vi "Read_queue_data.vi"(0 "Queue DVR in":refnum<data-value>, 11 "error in (no error)":errorcluster) -> (4 "Queue DVR out":refnum<data-value>, 6 "DATA":T1, 15 "error out":errorcluster)   [LabVIEW 2020, in "Data Communication Transmitter.lvlib" / "Queue.lvclass"]
uses:
  Classes/Children/Intra-Application/Children/With Data/Children/Queues/Queue.lvclass
  Classes/Children/Intra-Application/Children/With Data/Children/Queues/Queue.lvclass/Queue.ctl
  Accessors/Read/Read DATA.vi
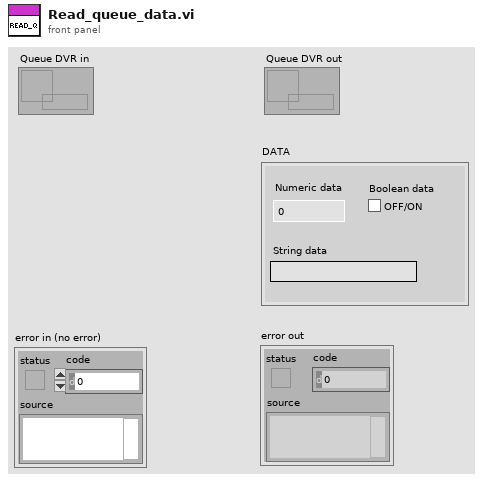
[diagram p1: front panel]
types:
  T1 = cluster{"Numeric data":dbl, "String data":string, "Boolean data":bool}
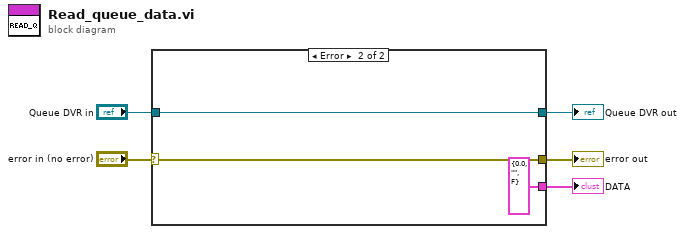
[diagram p0: block diagram]
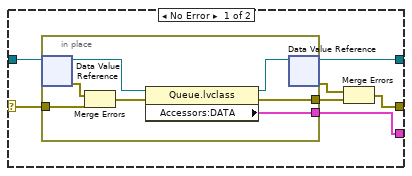
[diagram p2: hidden frame]
diagram:
  n1 = case shown="Error" "error in (no error)" {
    selector: "error in (no error)" -> [w11 w22]
    tunnel: [w8 w22] -> w4
    tunnel: "Queue DVR in" -> [w12 w21]
    tunnel: [w7 w21] -> w2
    tunnel: [w6 T1 {"Numeric data"=0.0, "String data"="", "Boolean data"=FALSE} ("Accessors:DATA")] -> w1
    frame No Error {
      n2 = in-place "In Place Element Structure" {
        in-place-border: [w17] -> w10
        in-place-border: w11 -> [w15]
        in-place-border: [w13] -> w6
        n3 = in-place-dvr #1(w12) -> (w16:refnum<class "Queue.lvclass">, w19:errorcluster)
        n4 = Merge Errors(w19, w15) -> (w18:errorcluster)
        n5 = property on="Property Node" class="Queue.lvclass"(reference=w16, error in=w18) -> (reference out=w14:refnum<class "Queue.lvclass">, error out=w17:errorcluster, "Accessors:DATA"=w13:T1)
        n6 = in-place-dvr #1(w14) -> (w7:refnum<data-value>, w9:errorcluster)
      }
      n7 = Merge Errors(w9, w10) -> (w8:errorcluster)
    }
    frame Error {
    }
  }
  "error out" <- w4
  "Queue DVR out" <- w2
  "DATA" <- w1
